vi "runtest.vi"(7 "httpRequestID":u32) -> ()   [LabVIEW 2011]
doc: "This VI is a state machine that can be ran from a Browser."
uses:
  server/database/Users/User Record.ctl
  <vilib>/wsapi/NI_WebServices.lvlib
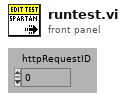
[diagram p1: front panel]
types:
  T1 = typedef "User Record.ctl" = cluster{"ixUser":i32, "sxUsername":string, "sLastName":string, "sFirstName":string, "sEmail":string, "sPassword":string, "tLoginTime":timestamp, "sLoginComputer":string, "fAdministrator":bool, "fRunSequences":bool, "fModifySequences":bool, "fRunScenarios":bool, "fModifyScenarios":bool, "fModifyTemplates":bool, "fModifyUsers":bool, "fModifyStations":bool, "fModifyFields":bool}
  T2 = typedef "Connection Refnum.ctl" = cluster{"Environment Handle":i32, "Connection Handle":i32}
  T3 = typedef "Keyed Array.ctl" = cluster{"keys":string[], "values":string[]}
  T4 = typedef "runtest User - Station.ctl" = cluster{"Username (\"\")":string, "Test Station IP (\"\")":string, "Test Station Name (\"\")":string, "Instruments on Station":T5[], "Step Associations":T6[]}
  T5 = typedef "Instrument Record.ctl" = cluster{"ixInstrument":i32, "sxInstrumentId":string, "sDriverId":string, "sDriverType":string, "sSerialNumber":string, "tLastCalibration":timestamp, "tCalibrationDue":timestamp, "sConfiguration":string}
  T6 = typedef "Step Association Record.ctl" = cluster{"ixStepAssociation":i32, "iStep":i32, "iStation":i32, "iInstrument":i32}
  T7 = typedef "Field Record.ctl" = cluster{"ixField":i32, "iSequenceOrder":i32, "sxFieldId":string, "sxSequenceId":string, "sDisplayName":string, "sValue":string, "sUnits":string, "nDataType":T8, "nNextItem":T9, "fSystem":bool, "fSystemValue":bool, "fRequired":bool, "fSetAtTest":bool, "fTestField":bool, "fDeleted":bool, "fIndexed":bool, "fFreeList":bool}
  T8 = typedef "Field DataTypes.ctl" = enum32{"text", "numeric", "list", "timestamp", "boolean"}
  T9 = typedef "Field NextItem.ctl" = enum32{"Reset", "Retain", "Auto-Increment"}
  T10 = typedef "Test Output.ctl" = cluster{"Status":string, "Message":string, "Results":string, "Abort All":bool, "Save Results?":bool, "Timing Metrics":string}
  T11 = cluster{"Sequence Fields with System Values":T7[], "Results":T10[]}
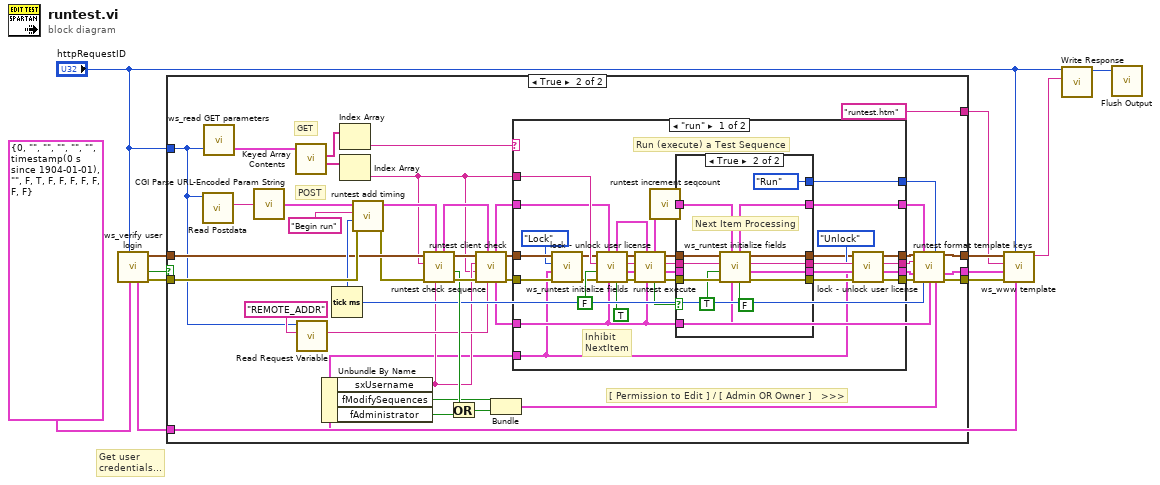
[diagram p0: block diagram]
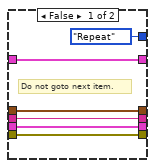
[diagram p3: hidden frame]
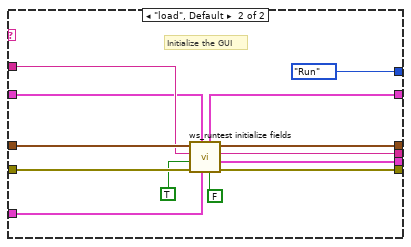
[diagram p4: hidden frame]
diagram:
  # "Get user \ncredentials..."
  n1 = call "ws_verify user login.vi"("Required Permisions"=T1 {"ixUser"=0, "sxUsername"="", "sLastName"="", "sFirstName"="", "sEmail"="", "sPassword"="", "tLoginTime"=timestamp(0 s since 1904-01-01), "sLoginComputer"="", "fAdministrator"=FALSE, "fRunSequences"=TRUE, "fModifySequences"=FALSE, "fRunScenarios"=FALSE, "fModifyScenarios"=FALSE, "fModifyTemplates"=FALSE, "fModifyUsers"=FALSE, "fModifyStations"=FALSE, "fModifyFields"=FALSE} ("User Record"), "httpRequestID"="httpRequestID") -> ("error out"=w12:errorcluster, "User Verified\nand Spartan\nAuthorized?"=w11:bool, "DB Connection Ref"=w10:T2, "User"=w4:T1)  [unwired: 6 in]
  n2 = case shown="True" w11 {
    tunnel: [w14 w26] -> w8
    tunnel: w10 -> [w13 w21]
    tunnel: w12 -> [w14 w35]
    tunnel: w4 -> [_ w15]
    tunnel: [_ "runtest.htm" ("Template (\"\")")] -> w5
    tunnel: [w13 w23] -> w6
    tunnel: [_ w22] -> w7
    tunnel: "httpRequestID" -> [_ w18]
    frame False {
    }
    frame True {
      # "[ Permission to Edit ] / [ Admin OR Owner ]   >>>"
      # "GET"
      # "POST"
      n3 = call <vilib>:"Read Postdata.vi"("httpRequestID"=w18) -> ("postdata"=w19:string)  [unwired: 8 in, 2 out]
      n4 = call "ws_read GET parameters.vi"("httpRequestID"=w18) -> ("GET query params"=w24:T3)  [unwired: 2 in]
      n5 = call <vilib>:"CGI Parse URL-Encoded Param String.vi"("url-encoded param string"=w19) -> ("params"=w38:T3)
      n6 = call <vilib>:"Keyed Array Contents.vi"("array in"=w24) -> ("values"=w54:string[], "keys"=w53:string[])  [unwired: 4 in, 1 out]
      n7 = call <vilib>:"Read Request Variable.vi"("variable name"="REMOTE_ADDR" ("key"), "httpRequestID"=w18) -> ("value"=w30:string)  [unwired: 7 in, 2 out]
      n8 = Unbundle By Name(w15) -> ("sxUsername"=w27:string, "fModifySequences"=w29:bool, "fAdministrator"=w28:bool)
      n9 = Tick Count (ms)() -> (millisecond timer value=w32:u32)
      n10 = Index Array(array=w53) -> (element=w52:string)  [unwired: 1 in]
      n11 = Index Array(array=w54) -> (element=w16:string)  [unwired: 1 in]
      n12 = call "runtest add timing.vi"("error in (no error)"=w35, "Start Tick, ms (0)"=w32, "Function (\"\")"="Begin run" ("Function (\"\")"), "POST (empty)"=w38) -> ("error out"=w20:errorcluster, "POST out"=w37:T3)  [unwired: 6 out]
      n13 = call "runtest check sequence.vi"("username (\"\")"=w27, "POST (empty)"=w37, "error in (no error)"=w20, "Sequence ID (\"\")"=w16, "Connection Refnum"=w21) -> ("error out"=w44:errorcluster, "Sequence Owner?"=w42:bool, "Connection Refnum"=w45:T2, "POST out"=w40:T3)  [unwired: 3 out]
      n14 = Or(x=w42, y=w28) -> (x .or. y?=w43:bool)
      n15 = call "runtest client check.vi"("Client IP or Domain Name (\"\")"=w30, "POST (empty)"=w40, "error in (no error)"=w44, "sxSequenceId"=w16, "Username (\"\")"=w27, "Connection Refnum"=w45) -> ("error out"=w46:errorcluster, "Connection Refnum"=w47:T2, "User/Station"=w17:T4, "POST out"=w39:T3)  [unwired: 2 out]
      n16 = Bundle("fModifySequences"=w29, w43) -> (w41:cluster{"fModifySequences":bool, bool})  [unwired: 1 out]
      n17 = case shown="\"run\"" w52 {
        tunnel: w46 -> [w66 w118]
        tunnel: w16 -> [w73 w115]
        tunnel: [w58 w113] -> w33
        tunnel: w47 -> [w65 w116]
        tunnel: [w59 w114] -> w50
        tunnel: w39 -> [w70 w108]
        tunnel: w17 -> [w72 w117]
        tunnel: [w82 enum16{"Run", "Repeat"}."Run" ("Button Name (Run)")] -> w31
        tunnel: [w81 w111] -> w49
        tunnel: [w80 w110] -> w48
        tunnel: [w79 w107] -> w34
        tunnel: w15 -> [w55 _]
        frame "run" {
          # "Inhibit \nNextItem"
          # "Run (execute) a Test Sequence"
          n18 = call "lock - unlock user license.vi"("error in (no error)"=w66, "User Record"=w55, "Action"=enum16{"Lock", "Unlock"}."Lock", "Connection Refnum"=w65) -> ("error out"=w63:errorcluster, "Connection Refnum"=w64:T2)  [unwired: 6 out]
          n19 = call "ws_runtest initialize fields.vi"("Process SPARTAN SN (F)"=TRUE, "User/Station"=w72, "POST (empty)"=w70, "error in (no error)"=w63, "ProcessNextItem? (f)"=FALSE, "Test Sequence ID"=w73, "Connection Refnum"=w64) -> ("error out"=w75:errorcluster, "Fields / Results"=w69:T11, "dup Test Sequence ID"=w74:string, "Connection Refnum"=w76:T2, "POST out"=w68:T3)
          n20 = call "runtest execute.vi"("User/Station"=w72, "POST (empty)"=w68, "error in (no error)"=w75, "Fields / Results"=w69, "Test Sequence ID"=w74, "Connection Refnum"=w76) -> ("error out"=w86:errorcluster, "Updated Fields / Results"=w78:T11, "dup Test Sequence ID"=w83:string, "Connection Refnum"=w85:T2, "Next Item?"=w84:bool, "POST out"=w67:T3)
          n21 = call "runtest increment seqcount.vi"("POST (empty)"=w67) -> ("new POST"=w77:T3)  [unwired: 3 out]
          n22 = case shown="True" w84 {
            tunnel: w86 -> [w92 w105]
            tunnel: [w92 w104] -> w57
            tunnel: [enum16{"Run", "Repeat"}."Repeat" ("Button Name (Run)") enum16{"Run", "Repeat"}."Run" ("Button Name (Run)")] -> w82
            tunnel: w77 -> [w88 w95]
            tunnel: w72 -> [_ w102]
            tunnel: w85 -> [w90 w101]
            tunnel: [w90 w100] -> w60
            tunnel: w83 -> [w89 w99]
            tunnel: [w87 w98] -> w80
            tunnel: [w89 w97] -> w81
            tunnel: [w88 w94] -> w79
            tunnel: w78 -> [w87 _]
            frame False {
              # "Do not goto next item."
            }
            frame True {
              # "Next Item Processing"
              n23 = call "ws_runtest initialize fields.vi"("Process SPARTAN SN (F)"=FALSE, "User/Station"=w102, "POST (empty)"=w95, "error in (no error)"=w105, "ProcessNextItem? (f)"=TRUE, "Test Sequence ID"=w99, "Connection Refnum"=w101) -> ("error out"=w104:errorcluster, "Fields / Results"=w98:T11, "dup Test Sequence ID"=w97:string, "Connection Refnum"=w100:T2, "POST out"=w94:T3)
            }
          }
          n24 = call "lock - unlock user license.vi"("error in (no error)"=w57, "User Record"=w55, "Action"=enum16{"Lock", "Unlock"}."Unlock", "Connection Refnum"=w60) -> ("error out"=w58:errorcluster, "Connection Refnum"=w59:T2)  [unwired: 6 out]
        }
        frame "load", Default {
          # "Initialize the GUI"
          n25 = call "ws_runtest initialize fields.vi"("Process SPARTAN SN (F)"=FALSE, "User/Station"=w117, "POST (empty)"=w108, "error in (no error)"=w118, "ProcessNextItem? (f)"=TRUE, "Test Sequence ID"=w115, "Connection Refnum"=w116) -> ("error out"=w113:errorcluster, "Fields / Results"=w110:T11, "dup Test Sequence ID"=w111:string, "Connection Refnum"=w114:T2, "POST out"=w107:T3)
        }
      }
      n26 = call "runtest format template keys.vi"("Connection Refnum"=w50, "POST (empty)"=w34, "User Action (Run)"=w31, "Test Sequence ID"=w49, "Fields / Results"=w48, "error in (no error)"=w33, "Timer"=w32, "User/Station"=w17, "Run Permissions"=w41) -> ("Connection Refnum"=w23:T2, "Template Keys"=w22:T3, "error out"=w26:errorcluster)  [unwired: 4 in]
    }
  }
  n27 = call "ws_www template.vi"("User"=w4, "httpRequestID"="httpRequestID", "error in (no error)"=w8, "Template Keys (empty)"=w7, "Template (\"\")"=w5, "DB Connection Ref"=w6) -> ("HTTP Template Content"=w2:string)  [unwired: 5 in]
  n28 = call <vilib>:"Write Response.vi"("response string"=w2, "httpRequestID"="httpRequestID") -> ("httpRequestID out"=w1:u32)  [unwired: 8 in, 1 out]
  n29 = call <vilib>:"Flush Output.vi"("httpRequestID"=w1) -> ()  [unwired: 9 in, 2 out]
